vi "multiply.vi"   [LabVIEW 2023, in "LabGRAD.lvlib" / "Value.lvclass"]
uses:
  LabVIEW projects/LabGRAD/Value/Value.lvclass
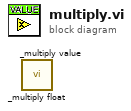
[diagram p0: block diagram]
diagram:
  n1 = call "_multiply float.vi"() -> ()  [unwired: 9 in, 3 out]
  n2 = call "_multiply value.vi"() -> ()  [unwired: 9 in, 3 out]
